vi "Stub.vi"(11 "Test Case In":refnum<class "Tests Event MessengerM.lvclass">) -> (0 "error out":errorcluster, 3 "Test Case Out":refnum<class "Tests Event MessengerM.lvclass">)   [LabVIEW 2020, in "Tests Event MessengerM.lvclass"]
uses:
  Tests Event MessengerM.lvclass
  C:/Program Files/National Instruments/LabVIEW 2026/vi.lib/Astemes/LUnit/Test Case.lvclass
  <vilib>/Astemes/LUnit/Test Case.lvclass/Test Case.ctl
  <vilib>/Astemes/LUnit/Test Case.lvclass
  491b4e49-c02a-443b-afb3-916e434634ff.vi
  099056c1-c7d2-4627-a7a6-09ded4223da2.vi
  72f7fc23-326d-46f3-a27b-8b3b109c1f1e.vi
  ae66f11c-5a1c-45ab-9a1b-6bf0d8107b45.vi
  680f33a2-57b4-46d7-8c5a-e6ca766f22c6.vi
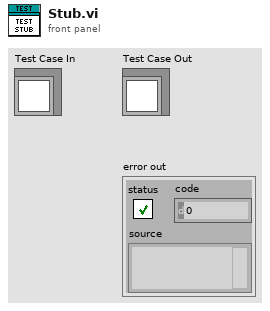
[diagram p1: front panel]
types:
  T1 = typedef "Event MessengerM-i32.lvlib/))Channel.ctl" = refnum<queue>
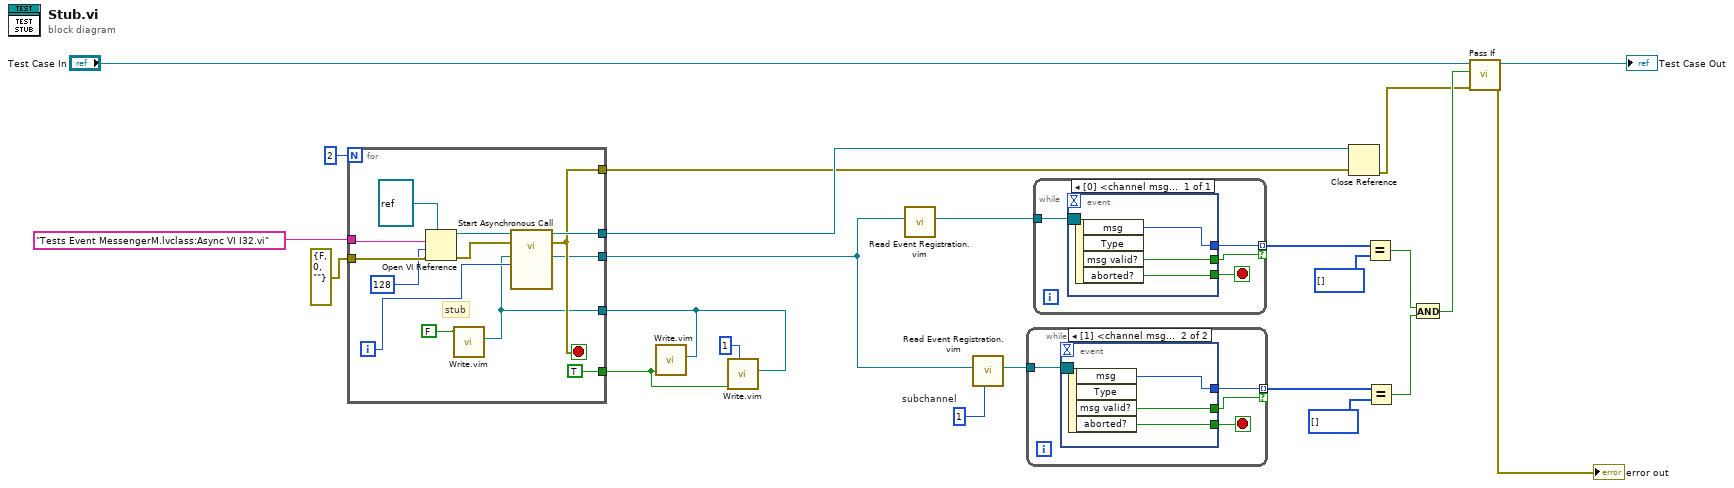
[diagram p0: block diagram]
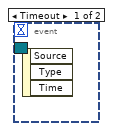
[diagram p2: hidden frame]
diagram:
  w1 = 1  # subchannel
  n1 = for {
    N: 2 -> [_]
    tunnel: "Tests Event MessengerM.lvclass:Async VI I32.vi" -> [w36]
    tunnel: errorcluster {"status"=FALSE, "code"=0, "source"=""} ("error constant") -> [w32]
    tunnel: [w31] -> w16
    tunnel: [w29] -> w14
    tunnel: [w27] -> w5
    tunnel: [w25] -> w4
    tunnel: [TRUE ("abort sub (F)")] -> w2
    i -> [w28]
    stop <- w29 stop-if-true
    # "stub"
    n2 = Open VI Reference(type specifier VI Refnum (for type only)=refnum<vi> refnum, vi path=w36, options=128, error in (no error)=w32) -> (vi reference=w34:refnum<vi>, error out=w33:errorcluster)  [unwired: 2 in]
    n3 = call "Write.vim"("message valid? (T)"=FALSE) -> ("channel"=w25:T1)  [unwired: 9 in, 1 out]
    n4 = call-by-ref "Start Asynchronous Call"(reference=w34, error in=w33, "subchannel (0)"=w28, "channel"=w25) -> (reference out=w31:refnum<vi>, error out=w29:errorcluster, "another channel"=w27:T1)  [unwired: 9 in]
  }
  n5 = call "Write.vim"("channel"=w4, "abort sub (F)"=w2) -> ()  [unwired: 9 in, 1 out]
  n6 = call "Write.vim"("channel"=w4, "subchannel"=1 ("subchannel (0)"), "abort sub (F)"=w2) -> ()  [unwired: 8 in, 1 out]
  n7 = call "Read Event Registration.vim"("channel"=w5) -> ("event registration refnum"=w7:refnum<event-registration>)  [unwired: 10 in]
  n8 = call "Read Event Registration.vim"("subchannel"=w1, "channel"=w5) -> ("event registration refnum"=w6:refnum<event-registration>)  [unwired: 9 in]
  n9 = while {
    tunnel: w6 -> [w40]
    tunnel: [w39] -> w12 mode=indexing if=w37
    stop <- w38 stop-if-true
    n10 = event shown="[1] <channel msg>: User Event" {
      selector: w40 -> [_ _]
      dyn-events: _ -> [_ _]
      timeout: _ -> [_ _]
      tunnel: [_ w43] -> w39
      tunnel: [_ w42] -> w38
      tunnel: [_ w41] -> w37
      event Timeout {
        n11 = event-data() -> ()  [unwired: 1 in, 3 out]
      }
      event User Event {
        n12 = event-data() -> ("msg"=w43:i32, "msg valid?"=w41:bool, "aborted?"=w42:bool)  [unwired: 1 in, 1 out]
      }
    }
  }
  n13 = while {
    tunnel: w7 -> [w47]
    tunnel: [w46] -> w13 mode=indexing if=w44
    stop <- w45 stop-if-true
    n14 = event shown="[0] <channel msg>: User Event" {
      selector: w47 -> [_]
      dyn-events: _ -> [_]
      timeout: _ -> [_]
      tunnel: [w50] -> w46
      tunnel: [w49] -> w45
      tunnel: [w48] -> w44
      event User Event {
        n15 = event-data() -> ("msg"=w50:i32, "msg valid?"=w48:bool, "aborted?"=w49:bool)  [unwired: 1 in, 1 out]
      }
    }
  }
  n16 = Close Reference(reference=w16, error in (no error)=w14) -> (error out=w15:errorcluster)
  n17 = Equal?(x=w13, y=i32[] []) -> (x = y?=w9:bool)
  n18 = Equal?(x=w12, y=i32[] []) -> (x = y?=w8:bool)
  n19 = And(x=w9, y=w8) -> (x .and. y?=w20:bool)
  n20 = call <vilib>:"Pass If.vi"("error in (no error)"=w15, "Pass?"=w20, "LUnit Test Case In"="Test Case In") -> ("error out"=→"error out":errorcluster, "LUnit Test Case Out"=→"Test Case Out":refnum<class "Tests Event MessengerM.lvclass">)  [unwired: 7 in]
